vi "New MC TDMS.vi"() -> (0 "error out":errorcluster, 3 "Refnum out":refnum<k34>)   [LabVIEW 2014]
uses:
  Global Data.vi
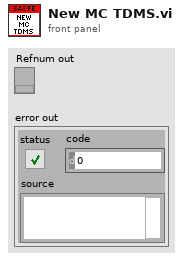
[diagram p1: front panel]
types:
  T1 = enum16{"open", "open or create", "create or replace", "create", "open (read-only)"}
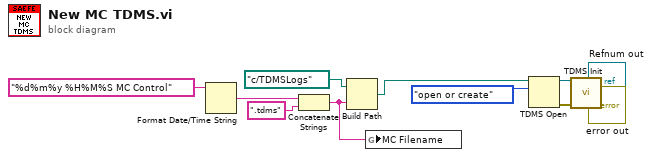
[diagram p0: block diagram]
diagram:
  n1 = Format Date/Time String(time format string (%c)="%d%m%y %H%M%S MC Control") -> (date/time string=w3:string)  [unwired: 2 in]
  n2 = Concatenate Strings(w3, ".tdms" ("string")) -> (w11:string)
  n3 = Build Path(base path=path "c:/TDMSLogs", name or relative path=w11) -> (appended path=w2:path)
  n4 = global write "Global Data.vi" "MC Filename"(w11) -> ()
  n5 = TDMS Open(10:T1."open or create" ("operation (0:open)"), 11:w2) -> (0:w8:errorcluster, 3:w7:refnum<k34>)  [unwired: 5 in]
  n6 = call "TDMS Init.vi"("error in (no error)"=w8, "tdms file"=w7) -> ("error out"=→"error out":errorcluster, "tdms file out"=→"Refnum out":refnum<k34>)  [unwired: 8 in]
